vi "FV_motor_get.vi"(6 "delay  (sec)":dbl=0.1 caption="Delay Time (s)", 7 "n_try":i8=1, 8 "error in":errorcluster, 10 "command":string="IP", 11 "VISA in":refnum<visa-resource-name>) -> (0 "error out":errorcluster, 1 "return_bytes":u32, 2 "return":string, 3 "VISA out":refnum<visa-resource-name>)   [LabVIEW 2019]
panel:
  out "return_i":string
  out "i":i32
  out "bytes":u32
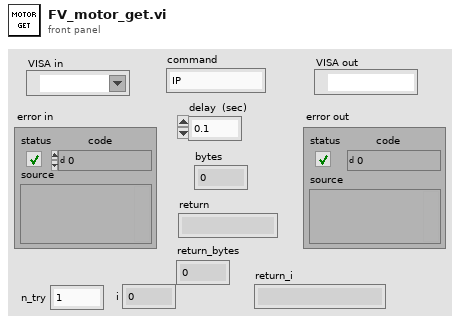
[diagram p1: front panel]
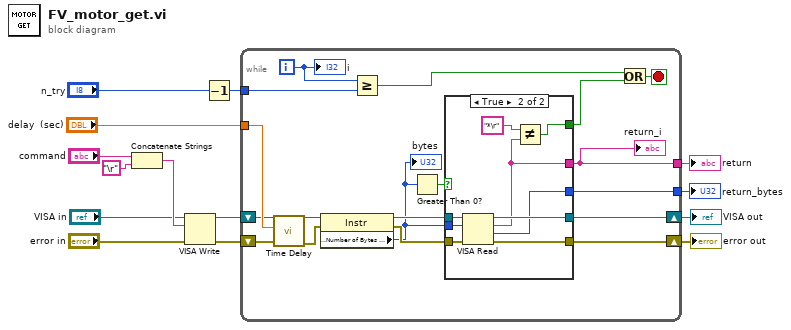
[diagram p0: block diagram]
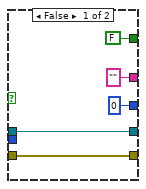
[diagram p2: hidden frame]
diagram:
  n1 = Concatenate Strings("command", "\r") -> (w14:string)
  n2 = VISA Write(VISA resource name="VISA in", write buffer=w14, error in (no error)="error in") -> (VISA resource name out=w7:refnum<visa-resource-name>, error out=w10:errorcluster)  [unwired: 1 out]
  n3 = Decrement(x="n_try") -> (x-1=w2:i8)
  n4 = while {
    tunnel: "delay  (sec)" -> [w30]
    tunnel: [w18] -> w4
    shift-right: [w25] -> w6
    shift-left: w10 -> [w31]
    shift-right: [w24] -> w5
    shift-left: w7 -> [w29]
    tunnel: w2 -> [w22]
    tunnel: [w15] -> w1
    i -> [w23]
    stop <- w21 stop-if-true
    n5 = call "Time Delay"("error in (no error)"=w31, "Delay Time (s)"=w30) -> ("error out"=w28:errorcluster)  [unwired: 9 in]
    n6 = property class="Instr"(reference=w29, error in=w28) -> (reference out=w27:refnum<visa-resource-name>, error out=w26:errorcluster, "Serial Settings:Number of Bytes at Serial Port"=w16:u32)
    "bytes" <- w16
    n7 = Greater Or Equal?(x=w23, y=w22) -> (x >= y?=w20:bool)
    n8 = Greater Than 0?(x=w16) -> (x > 0?=w17:bool)
    n9 = case shown="True" w17 {
      tunnel: w27 -> [w34 w45]
      tunnel: w26 -> [w33 w44]
      tunnel: w16 -> [_ w43]
      tunnel: [w33 w42] -> w25
      tunnel: [w34 w41] -> w24
      tunnel: [FALSE w40] -> w19
      tunnel: ["" ("read buffer") w39] -> w18
      tunnel: [u32 0 ("return count") w37] -> w15
      frame False {
      }
      frame True {
        n10 = VISA Read(VISA resource name=w45, byte count=w43, error in (no error)=w44) -> (VISA resource name out=w41:refnum<visa-resource-name>, read buffer=w39:string, return count=w37:u32, error out=w42:errorcluster)
        n11 = Not Equal?(x="*\r", y=w39) -> (x != y?=w40:bool)
      }
    }
    "return_i" <- w18
    n12 = Or(x=w20, y=w19) -> (x .or. y?=w21:bool)
    "i" <- w23
  }
  "VISA out" <- w5
  "error out" <- w6
  "return" <- w4
  "return_bytes" <- w1
